vi "Actor Core.vi"(8 "error in":errorcluster, 11 "Cooker Actor in":refnum<class "Cooker Actor.lvclass">) -> (0 "error out":errorcluster, 3 "Actor out":refnum<class "Actor.lvclass">)   [LabVIEW 2024, in "Cooker Actor.lvlib" / "Cooker Actor.lvclass"]
doc: "<p>(<strong>Filename</strong>: <span class=\"dnl\">Actor Framework.lvlib:Actor.lvclass:Actor Core.vi</span>)</p>\n<p>Receives messages to the actor, reacts to them, and initiates any error handling that may shut the actor down.</p>\n<p>Descendant classes may override this VI to append parallel tasks for the actor to complete while it handles messages. Overrides use the <a href=\"nihelplauncher://docs/csh?context=lvcore_glang_udclass\">Call Parent Class Method</a> node.</p>"
uses:
  Cooker Actor.lvclass
  Cooker Actor.lvclass/Cooker Actor.ctl
  <vilib>/ActorFramework/Actor/Actor.lvclass
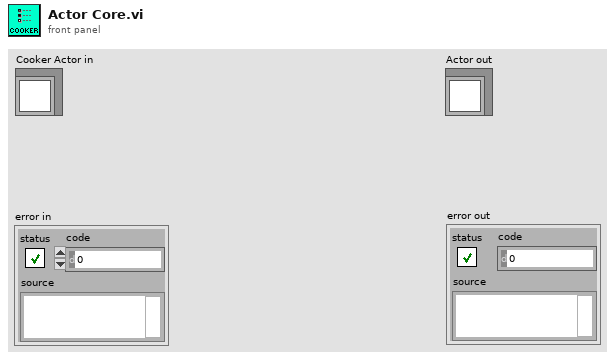
[diagram p1: front panel]
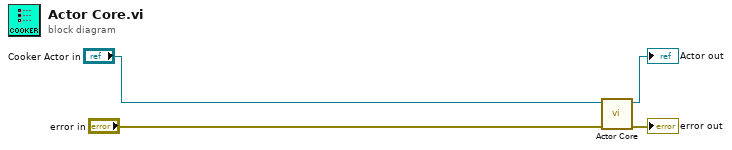
[diagram p0: block diagram]
diagram:
  n1 = call-parent "Actor Core.vi"("error in"="error in", "Actor in"="Cooker Actor in") -> ("error out"=→"error out":errorcluster, "Actor out"=→"Actor out":refnum<class "Actor.lvclass">)  [unwired: 8 in]
